vi "Set Last Pat.vi"(8 "error in (no error)":errorcluster, 9 "Last Pat":timestamp, 10 "ID":string, 11 "uService List in":refnum<class "uService List.lvclass">) -> (0 "error out":errorcluster, 3 "uService List out":refnum<class "uService List.lvclass">)   [LabVIEW 2026, in "TALOS.lvlib" / "Classes.lvlib" / "uService List.lvclass"]
uses:
  uService List.lvclass
  uService List.lvclass/uService List.ctl
  Ancestor/Ancestor/Ancestor.lvclass/Ancestor.ctl
  FGV/Error Memory/Get Error Description.vi
  Support VIs/Get PC name.vi
  Ancestor/Ancestor/Read ID.vi
  Support VIs/Get Class Name.vi
  <vilib>/Utility/error.llb/Clear Errors.vi
  FGV/Error Memory/Error Memory Core.vi
  <vilib>/AdvancedString/Delimited String to 1D String Array.vi
  <vilib>/AdvancedString/Delimited String to 1D String Array (string).vi
  Support VIs/Circus Root Path.vi
  FGV/Error Memory/Error Crt Lvl checker.vi
  FGV/Error Memory/Error Memory Core.vi/40c8088d-b597-4017-91af-faa98e00292e.vi
  FGV/Error Memory/Error Memory Core.vi/d4a3ab98-063c-4e44-b43d-fbdcfe6c2be2.vi
  Support VIs/Global Memory.vi
  <vilib>/Utility/LVClass/Get LV Class Name.vi
  Support VIs/Is in Packed Library.vi
  Support VIs/TALOS Root path.vi
  Support VIs/Read CSV worksheet.vi
  Support VIs/Global Constants.vi
  <vilib>/Utility/error.llb/General Error Handler.vi
  Ancestor/Ancestor/Ancestor.lvclass
  <vilib>/Comparison/Equal/Equal Functor/Equal Functor.lvclass
  TALOS.lvlib
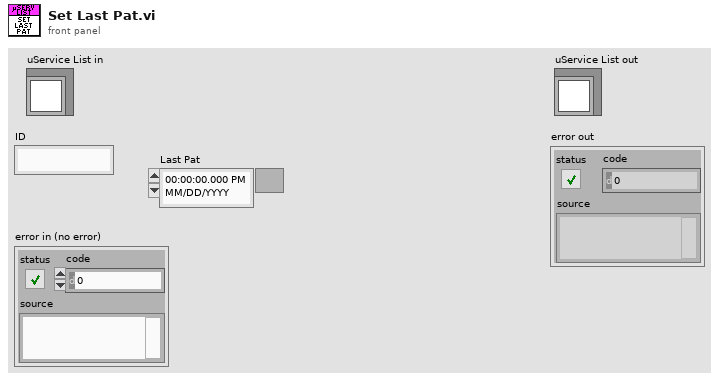
[diagram p1: front panel]
types:
  T1 = typedef "TALOS.lvlib/Classes.lvlib/uService List.lvclass/uService Properties.ctl" = cluster{"uService Queue":refnum<class "Message Enqueuer.lvclass">, "Last Pat":timestamp, "Online":bool, "Vi Ref":refnum<vi>, "Class name":string, "GUI":bool, "FP Items Refs Map":map{string, refnum<vi>}, "Remote GUI":bool, "Remote Window":refnum<vi>}
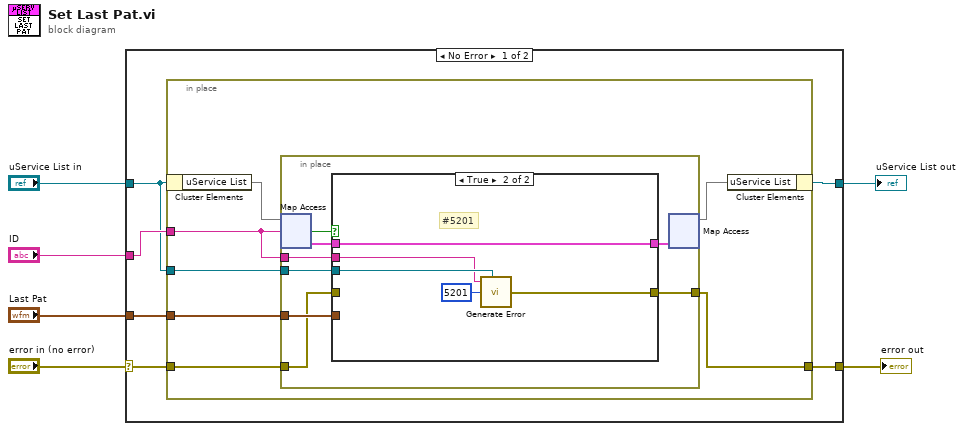
[diagram p0: block diagram]
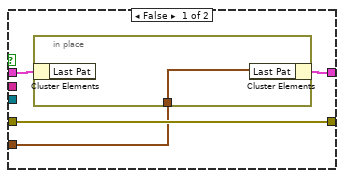
[diagram p2: hidden frame]
diagram:
  n1 = case shown="No Error" "error in (no error)" {
    selector: "error in (no error)" -> [w9 w39]
    tunnel: [w8 w39] -> w5
    tunnel: "uService List in" -> [w7 w38]
    tunnel: [w12 w38] -> w3
    tunnel: "ID" -> [w11 _]
    tunnel: "Last Pat" -> [w10 _]
    frame No Error {
      n2 = in-place {
        in-place-border: w11 -> [w13]
        in-place-border: w10 -> [w18]
        in-place-border: w9 -> [w17]
        in-place-border: [w16] -> w8
        in-place-border: w7 -> [w14]
        n3 = in-place-cluster #1(w7) -> ("uService List"=w19:map{string, T1})
        n4 = in-place "In Place Element Structure" {
          in-place-border: [w25] -> w16
          in-place-border: w18 -> [w23]
          in-place-border: w17 -> [w22]
          in-place-border: w14 -> [w21]
          in-place-border: w13 -> [w20]
          n5 = in-place-map #2(w19, w13) -> (w27:T1, w24:bool)  [unwired: 1 in]
          n6 = case shown="True" w24 {
            tunnel: w27 -> [w31 w37]
            tunnel: [w30 w37] -> w26
            tunnel: [w29 w35] -> w25
            tunnel: w22 -> [w29 _]
            tunnel: w23 -> [w28 _]
            tunnel: w21 -> [_ w34]
            tunnel: w20 -> [_ w33]
            frame False {
              n7 = in-place "In Place Element Structure" {
                in-place-border: w28 -> [w32]
                n8 = in-place-cluster #3(w31) -> ()  [unwired: 1 out]
                n9 = in-place-cluster #3("Last Pat"=w32) -> (w30:T1)
              }
            }
            frame True {
              # "#5201"
              n10 = call "Generate Error.vi"("Optional String"=w33, "Class"=w34, "Error Code"=5201) -> ("error out"=w35:errorcluster)  [unwired: 4 in]
            }
          }
          n11 = in-place-map #2(w26) -> (w15:map{string, T1})  [unwired: 1 in, 2 out]
        }
        n12 = in-place-cluster #1("uService List"=w15) -> (w12:refnum<class "uService List.lvclass">)
      }
    }
    frame Error {
    }
  }
  "error out" <- w5
  "uService List out" <- w3
